vi "Download Dependencies.vi"   [LabVIEW 2020]
uses:
  Binary Dependency Platform.ctl
  common/common.lvlib
types:
  T1 = typedef "Binary Dependency Platform.ctl" = enum16{"Windows Desktop x86", "Windows Desktop x64", "Linux Desktop x64", "NI Linux RT x64", "NI Linux RT armv7"}
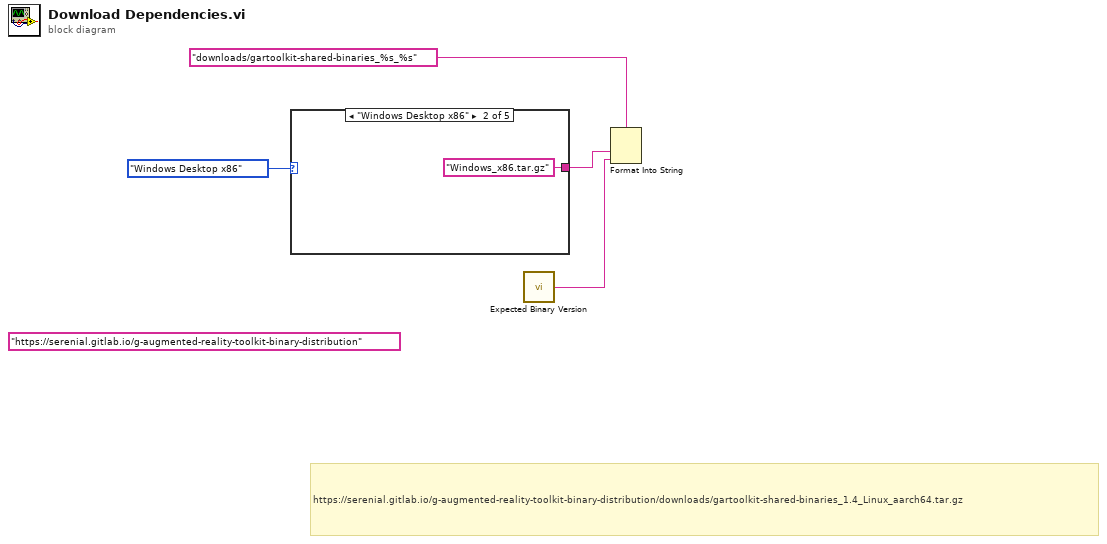
[diagram p0: block diagram]
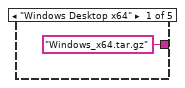
[diagram p2: hidden frame]
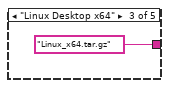
[diagram p3: hidden frame]
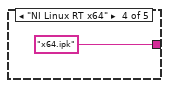
[diagram p4: hidden frame]
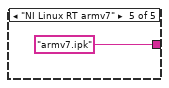
[diagram p5: hidden frame]
diagram:
  (unwired) "https://serenial.gitlab.io/g-augmented-reality-toolkit-binary-distribution"
  # "https://serenial.gitlab.io/g-augmented-reality-toolkit-binary-distribution/downloads/gartoolkit-shared-binaries_1.4_Linux_aarch64.tar.gz"
  n1 = case shown="\"Windows Desktop x86\"" Binary_Dependency_Platform."Windows Desktop x86" ("Platform") {
    tunnel: ["Windows_x64.tar.gz" "Windows_x86.tar.gz" "Linux_x64.tar.gz" "x64.ipk" "armv7.ipk"] -> w2
    frame "Windows Desktop x64" {
    }
    frame "Windows Desktop x86" {
    }
    frame "Linux Desktop x64" {
    }
    frame "NI Linux RT x64" {
    }
    frame "NI Linux RT armv7" {
    }
  }
  n2 = call "Expected Binary Version.vi"() -> ("Expected Version"=w1:string)
  n3 = Format Into String(format string="downloads/gartoolkit-shared-binaries_%s_%s", w2, w1) -> ()  [unwired: 2 in, 2 out]
